vi "Is command present in HLP answer.vi"   [LabVIEW 2026]
doc: "This VI checks whether the specified commands are present in the HLP? answer.\nIf Check HLP? is TRUE, HLP?.vi will be called to get HLP? information.\nIf Check HLP? is FALSE, a valid HLP? answer has to be provided in HLP answer."
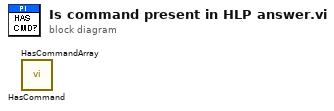
[diagram p0: block diagram]
diagram:
  n1 = call "HasCommand.vi"() -> ()  [unwired: 17 in, 3 out]
  n2 = call "HasCommandArray.vi"() -> ()  [unwired: 17 in, 3 out]
